vi "svc_Build dB Label (octave info).vi"(4 "width (-)":i16, 5 "number format":i16(ring) items=["Engineering", "Exponential", "Fractional", "Automatic"], 7 "include reference (T)":bool=TRUE, 9 "precision (1)":i16=1, 10 "octave info":T1={"standard"=enum."ANSI S1.11", "bandwidth"=enum."1 octave", "low band"=0, "high band"=0, "weighting filter"=0, "dB reference"=0.0, "dB On"=FALSE, "unit label"="", "channel name"="", "description"="", "engineering units"=1, "custom label"="", "spectrum type"=enum."magnitude", "spectral density"=FALSE, "filters settled"=FALSE} {"engineering units" items=["custom..."=0, "V"=1, "A"=21, "C"=30, "pC"=31, "s"=32, "-"=29, "Pa"=2, "N"=20, "g"=3, "m/s^2"=4, "m/s"=5, "m"=6, "mm/s"=12, "mm"=13, "micron/s"=14, "micron"=15, "in/s^2"=7, "in/s"=8, "in"=9, "mil/s"=10, "mil"=11, "rad/s^2"=16, "rad/s"=17, "rad"=18, "deg/s^2"=26, "deg/s"=27, "deg"=28, "RPM"=22, "cycle/s^2"=23, "Hz"=24, "cycle"=25, "strain"=19]; "dB reference" format="%.2e"; "weighting filter" items=["Linear", "A-weighting", "B-weighting", "C-weighting", "ITU-R 468-4", "Dolby", "CCITT", "C-message", "Wb", "Wc", "Wd", "We", "Wf", "Wh", "Wj", "Wk", "Wm", "AES17 20 kHz lowpass", "AES17 40 kHz lowpass", "AES17 20 kHz highpass", "AES17 40 kHz highpass"]}) -> (1 "dB reference [EU]":dbl format="%.2f", 2 "ref label":string, 3 "dB( )":string)   [LabVIEW 2017]
uses:
  <vilib>/addons/_NISVFA/_Shared subVIs/Controls/svc_Octave Info.ctl
  <vilib>/addons/_NISVFA/_Shared subVIs/Controls/svc_Octave Standard.ctl
  <vilib>/addons/_NISVFA/_Shared subVIs/Controls/svc_Weighting Filter Text Ring.ctl
  <vilib>/addons/_NISVFA/_Shared subVIs/Controls/svc_Engineering Units Text Ring.ctl
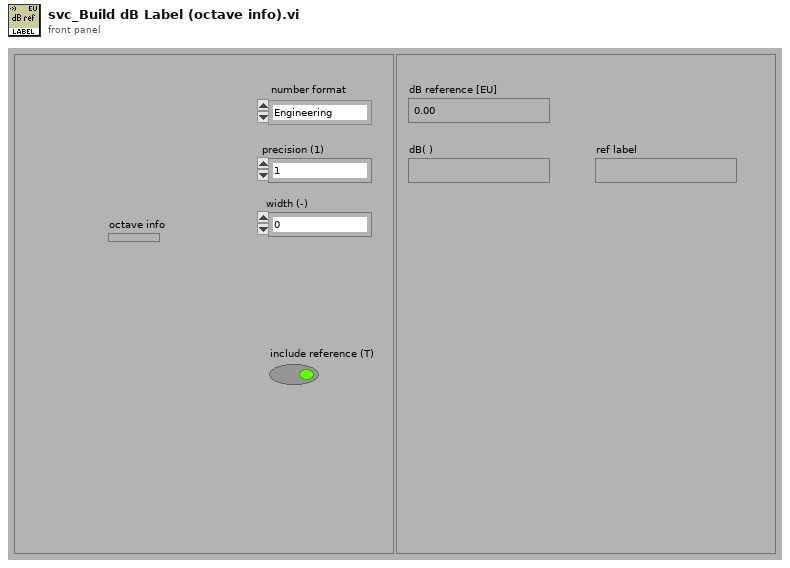
[diagram p1: front panel]
types:
  T1 = typedef "svc_Octave Info.ctl" = cluster{"standard":T2, "bandwidth":enum16{"1 octave", "1/3 octave", "1/6 octave", "1/12 octave", "1/24 octave"}, "low band":i32, "high band":i32, "weighting filter":T3, "dB reference":dbl, "dB On":bool, "unit label":string, "channel name":string, "description":string, "engineering units":T4, "custom label":string, "spectrum type":enum16{"power", "magnitude"}, "spectral density":bool, "filters settled":bool}
  T2 = typedef "svc_Octave Standard.ctl" = enum16{"ANSI S1.11", "IEC 61260"}
  T3 = typedef "svc_Weighting Filter Text Ring.ctl" = u16
  T4 = typedef "svc_Engineering Units Text Ring.ctl" = u16
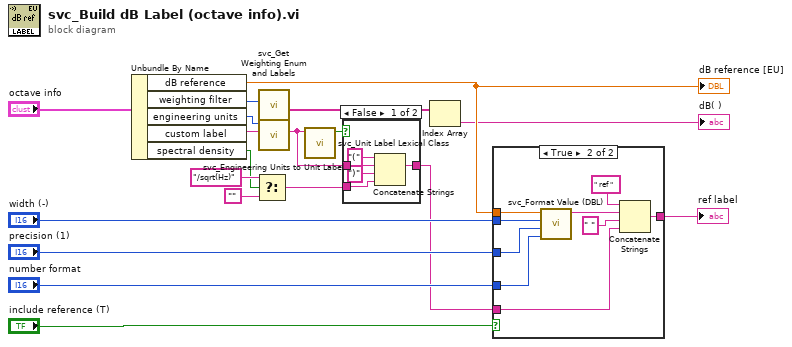
[diagram p0: block diagram]
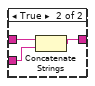
[diagram p2: hidden frame]
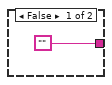
[diagram p3: hidden frame]
diagram:
  n1 = Unbundle By Name("octave info") -> ("dB reference"=w15:dbl, "weighting filter"=w2:T3, "engineering units"=w10:T4, "custom label"=w9:string, "spectral density"=w5:bool)
  "dB reference [EU]" <- w15
  n2 = Select(t="/sqrt(Hz)", s=w5, f="") -> (s? t:f=w6:string)
  n3 = call <vilib>:"svc_Get Weighting Enum and Labels.vi"("weighting filter"=w2) -> ("weighting subarray"=w3:string[])  [unwired: 7 in, 1 out]
  n4 = call <vilib>:"svc_Engineering Units to Unit Label.vi"("custom label"=w9, "engineering units"=w10) -> ("unit label"=w12:string)  [unwired: 8 in, 1 out]
  n5 = call <vilib>:"svc_Unit Label Lexical Class.vi"("unit label"=w12) -> ("letters only?"=w11:bool)  [unwired: 6 in]
  n6 = case shown="False" w11 {
    tunnel: w12 -> [w24 w27]
    tunnel: [w23 w25] -> w8
    tunnel: w6 -> [w20 w26]
    frame False {
      n7 = Concatenate Strings("(" ("string"), w24, ")" ("string"), w20) -> (w23:string)
    }
    frame True {
      n8 = Concatenate Strings(w27, w26) -> (w25:string)
    }
  }
  n9 = Index Array(array=w3) -> (element=→"dB( )":string)  [unwired: 1 in]
  n10 = case shown="True" "include reference (T)" {
    tunnel: ["" w37] -> w17
    tunnel: w15 -> [_ w33]
    tunnel: "number format" -> [_ w31]
    tunnel: w8 -> [_ w35]
    tunnel: "width (-)" -> [_ w30]
    tunnel: "precision (1)" -> [_ w29]
    frame False {
    }
    frame True {
      n11 = call <vilib>:"svc_Format Value (DBL).vi"("number format"=w31, "precision (1)"=w29, "width (-)"=w30, "dB reference"=w33) -> ("format string"=w32:string)  [unwired: 7 in]
      n12 = Concatenate Strings(" ref ", w32, " " ("Substring"), w35) -> (w37:string)
    }
  }
  "ref label" <- w17
